vi "SLSC CD Schema Path.vi"() -> (2 "SLSC CD Schema Path":string)   [LabVIEW 2020, in "VeriStand SLSC Scripting.lvlib"]
uses:
  VeriStand SLSC Scripting.lvlib
  NationalInstruments.VeriStand.SystemStorage
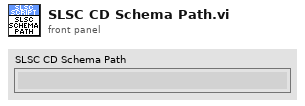
[diagram p1: front panel]
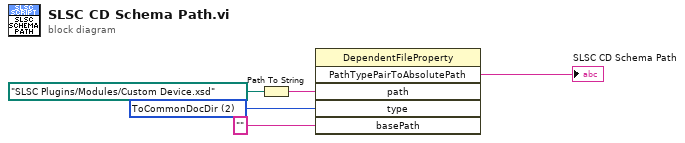
[diagram p0: block diagram]
diagram:
  w4 = 2 items=["Absolute", "Relative", "ToCommonDocDir", "ToApplicationDataDir"] ("type")
  n1 = Path To String(path=path "SLSC Plugins/Modules/Custom Device.xsd") -> (string=w1:string)
  n2 = invoke class="DependentFileProperty" method="PathTypePairToAbsolutePath"("path"=w1, "type"=w4, "basePath"="") -> ("PathTypePairToAbsolutePath"=→"SLSC CD Schema Path":string)  [unwired: 3 in, 5 out]
